vi "test_MonoFilterWheel.vi"(8 "error in":errorcluster, 11 "Monochromator in":refnum<class "Monochromator.lvclass">) -> (0 "error out":errorcluster, 3 "Monochromator out":refnum<class "Monochromator.lvclass">)   [LabVIEW 2023, in "horiba.test.lvlib"]
uses:
  Classes/Mono/Monochromator.lvclass
  C:/Projects/Horiba/horiba-labview-sdk/Source/Classes/GenericDevice/GenericDevice.lvclass
  520836cf-1509-4afe-994a-29c0f161cc02.vi
  db89a6f4-bc2a-445d-a728-0b1a27007309.vi
  00798782-67c5-400d-a46f-144718c20ccd.vi
  <vilib>/addons/_JKI Toolkits/Caraya/classes/Assert/Assert Equal Value_Variant.vi
  horiba.test.lvlib
  <vilib>/addons/_JKI Toolkits/Caraya/classes/Test/Test.lvclass
  <vilib>/addons/_JKI Toolkits/Caraya/classes/Assert/Assert.lvclass
  <userlib>/_OpenG.lib/lvdata/lvdata.llb/openg_variant.lvlib
panel:
  # "Connector Pane"
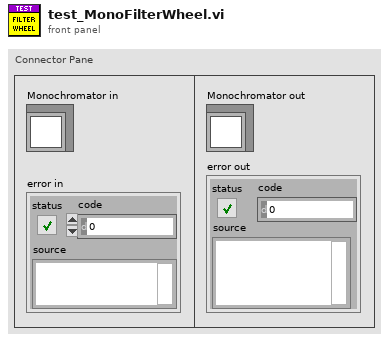
[diagram p1: front panel]
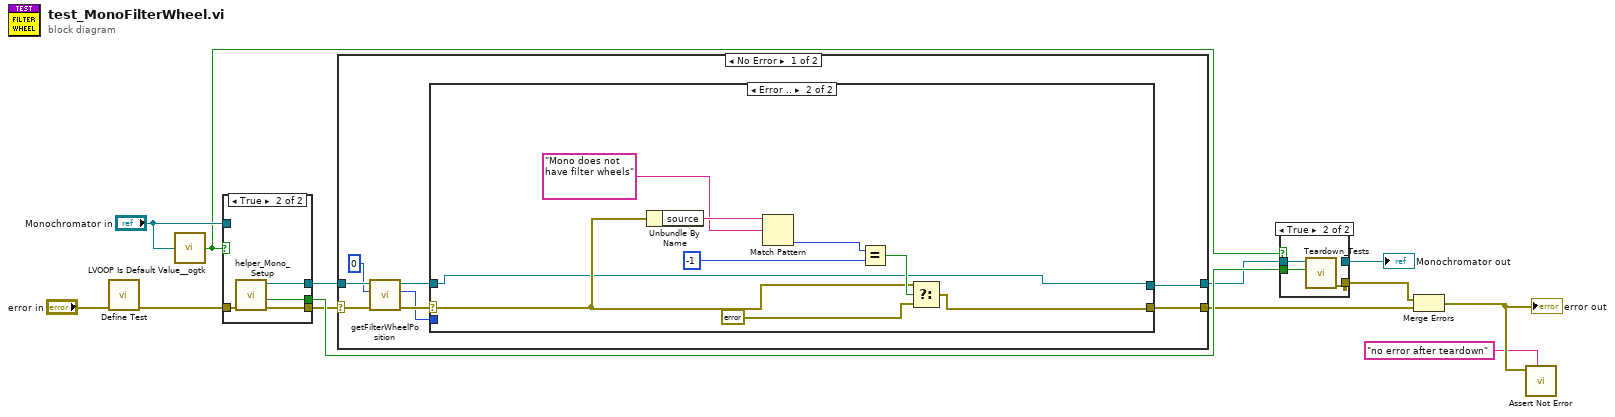
[diagram p0: block diagram]
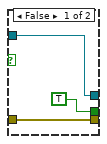
[diagram p3: hidden frame]
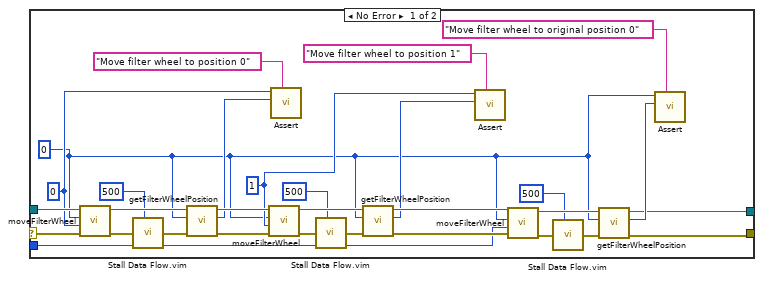
[diagram p4: hidden frame]
diagram:
  n1 = call <vilib>:"Define Test.vi"("error in (no error)"="error in") -> ("error out"=w7:errorcluster)  [unwired: 9 in, 1 out]
  n2 = call <userlib>:"LVOOP Is Default Value__ogtk.vi"("Object"="Monochromator in") -> ("Is Default Value?"=w8:bool)
  n3 = case shown="True" w8 {
    tunnel: w7 -> [w15 w20]
    tunnel: [w15 w19] -> w2
    tunnel: [w16 w18] -> w5
    tunnel: [TRUE ("Module Was Already Running?") w17] -> w10
    tunnel: "Monochromator in" -> [w16 _]
    frame False {
    }
    frame True {
      n4 = call "helper_Mono_Setup.vi"("error in"=w20) -> ("error out"=w19:errorcluster, "Module Was Already Running?"=w17:bool, "Monochromator out"=w18:refnum<class "Monochromator.lvclass">)  [unwired: 7 in, 1 out]
    }
  }
  n5 = case shown="No Error" w2 {
    selector: w2 -> [w28 w69]
    tunnel: [w21 w68] -> w4
    tunnel: w5 -> [w27 w68]
    tunnel: [w24 w69] -> w1
    frame No Error {
      n6 = call "getFilterWheelPosition.vi"("error in (no error)"=w28, "locationId"=0, "Monochromator in"=w27) -> ("error out"=w25:errorcluster, "position"=w22:i32, "Monochromator out"=w23:refnum<class "Monochromator.lvclass">)  [unwired: 6 in]
      n7 = case shown="Error .." w25 {
        selector: w25 -> [w46 w62]
        tunnel: [w40 w60] -> w24
        tunnel: w23 -> [w48 w59]
        tunnel: w22 -> [w47 _]
        tunnel: [w29 w59] -> w21
        frame No Error {
          w36 = 1 ("position")
          w43 = 0 ("position")
          w33 = 0 ("position")
          n8 = call "moveFilterWheel.vi"("error in (no error)"=w46, "position"=w43, "locationId"=w33, "Monochromator in"=w48) -> ("error out"=w57:errorcluster, "Monochromator out"=w58:refnum<class "Monochromator.lvclass">)  [unwired: 4 in, 2 out]
          n9 = call "Stall Data Flow.vim"("value in"=w57, "milliseconds to wait"=u32 500) -> ("value out"=w45:errorcluster)  [unwired: 1 out]
          n10 = call "getFilterWheelPosition.vi"("error in (no error)"=w45, "locationId"=w33, "Monochromator in"=w58) -> ("error out"=w55:errorcluster, "position"=w42:i32, "Monochromator out"=w56:refnum<class "Monochromator.lvclass">)  [unwired: 6 in]
          n11 = call "moveFilterWheel.vi"("error in (no error)"=w55, "position"=w36, "locationId"=w33, "Monochromator in"=w56) -> ("error out"=w53:errorcluster, "Monochromator out"=w54:refnum<class "Monochromator.lvclass">)  [unwired: 4 in, 2 out]
          n12 = call-poly <vilib>:"Assert.vi"("Label"="Move filter wheel to position 0", "Y"=w42, "X"=w43) -> ()  [unwired: 7 in, 2 out]
          n13 = call "Stall Data Flow.vim"("value in"=w53, "milliseconds to wait"=u32 500) -> ("value out"=w39:errorcluster)  [unwired: 1 out]
          n14 = call "getFilterWheelPosition.vi"("error in (no error)"=w39, "locationId"=w33, "Monochromator in"=w54) -> ("error out"=w51:errorcluster, "position"=w35:i32, "Monochromator out"=w52:refnum<class "Monochromator.lvclass">)  [unwired: 6 in]
          n15 = call-poly <vilib>:"Assert.vi"("Label"="Move filter wheel to position 1", "Y"=w35, "X"=w36) -> ()  [unwired: 7 in, 2 out]
          n16 = call "moveFilterWheel.vi"("error in (no error)"=w51, "position"=w47, "locationId"=w33, "Monochromator in"=w52) -> ("error out"=w49:errorcluster, "Monochromator out"=w50:refnum<class "Monochromator.lvclass">)  [unwired: 4 in, 2 out]
          n17 = call "Stall Data Flow.vim"("value in"=w49, "milliseconds to wait"=u32 500) -> ("value out"=w31:errorcluster)  [unwired: 1 out]
          n18 = call "getFilterWheelPosition.vi"("error in (no error)"=w31, "locationId"=w33, "Monochromator in"=w50) -> ("error out"=w40:errorcluster, "position"=w32:i32, "Monochromator out"=w29:refnum<class "Monochromator.lvclass">)  [unwired: 6 in]
          n19 = call-poly <vilib>:"Assert.vi"("Label"="Move filter wheel to original position 0", "Y"=w32, "X"=w33) -> ()  [unwired: 7 in, 2 out]
        }
        frame Error {
          n20 = Unbundle By Name(w62) -> ("source"=w67:string)
          n21 = Match Pattern(string=w67, regular expression="Mono does not have filter wheels") -> (offset past match=w65:i32)  [unwired: 1 in, 3 out]
          n22 = Equal?(x=w65, y=-1) -> (x = y?=w63:bool)
          n23 = Select(t=w62, s=w63, f=errorcluster {"status"=FALSE, "code"=0, "source"=""}) -> (s? t:f=w60:errorcluster)
        }
      }
    }
    frame Error {
    }
  }
  n24 = case shown="True" w8 {
    tunnel: w4 -> [w70 w73]
    tunnel: [_ w72] -> w6
    tunnel: w10 -> [_ w71]
    tunnel: [w70 _] -> w3
    frame False {
    }
    frame True {
      n25 = call "Teardown_Tests.vi"("Module Was Already Running?"=w71, "horiba.lvlib:GenericDevice"=w73) -> ("error out"=w72:errorcluster)  [unwired: 8 in, 1 out]
    }
  }
  "Monochromator out" <- w3
  n26 = Merge Errors(w6, w1) -> (w12:errorcluster)
  "error out" <- w12
  n27 = call <vilib>:"Assert Not Error.vi"("Label"="no error after teardown", "Not Error?"=w12) -> ()  [unwired: 8 in, 2 out]
